vi "Write Phase.vi"(8 "error in (no error)":errorcluster, 10 "Phase":dbl, 11 "Analog Waveform in":refnum<class "Analog Waveform.lvclass">) -> (0 "error out":errorcluster, 3 "Analog Waveform out":refnum<class "Analog Waveform.lvclass">)   [LabVIEW 2020, in "Analog Waveform.lvclass"]
uses:
  Analog Waveform.lvclass
  Analog Waveform.lvclass/Analog Waveform.ctl
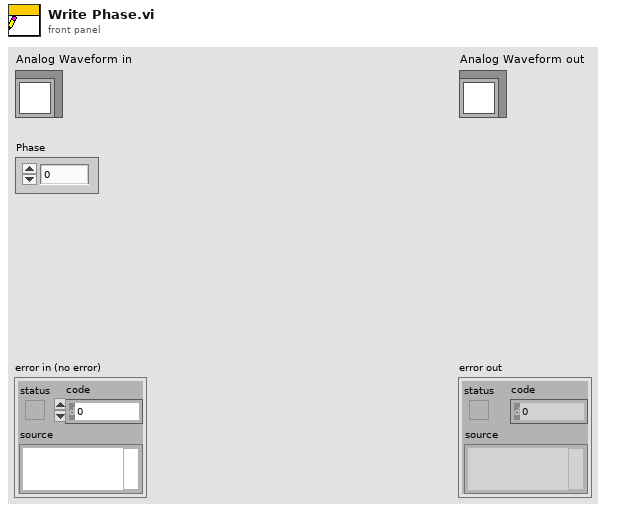
[diagram p1: front panel]
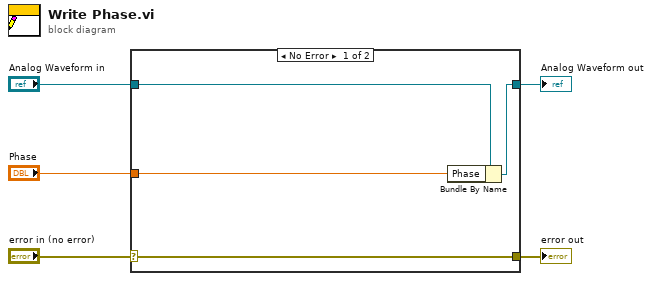
[diagram p0: block diagram]
diagram:
  n1 = case shown="No Error" "error in (no error)" {
    selector: "error in (no error)" -> [w9 w10]
    tunnel: [w9 w10] -> w4
    tunnel: [w7 w11] -> w2
    tunnel: "Analog Waveform in" -> [w8 w11]
    tunnel: "Phase" -> [w6 _]
    frame No Error {
      n2 = Bundle By Name(cluster=w8, "Phase"=w6) -> (w7:refnum<class "Analog Waveform.lvclass">)
    }
    frame Error {
    }
  }
  "error out" <- w4
  "Analog Waveform out" <- w2
